vi "Simulation LV2G.vi"(6 "Operation (Get)":T1=enum."Get", 8 "error in (no error)":errorcluster, 11 "Simulation?":bool) -> (0 "error out":errorcluster, 3 "Simulation? out":bool)   [LabVIEW 2016]
uses:
  Typedefs/LV2G Operation.ctl
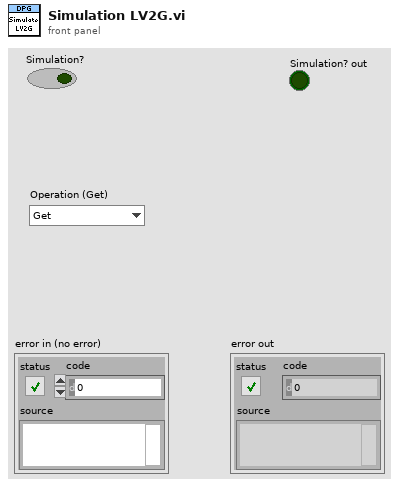
[diagram p1: front panel]
types:
  T1 = typedef "LV2G Operation.ctl" = enum16{"Initialize", "Set", "Get", "Close"}
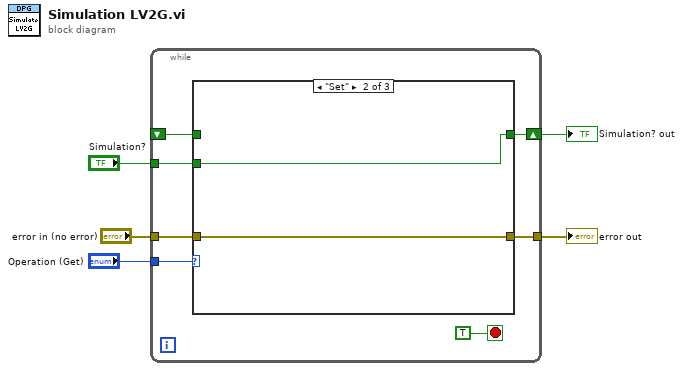
[diagram p0: block diagram]
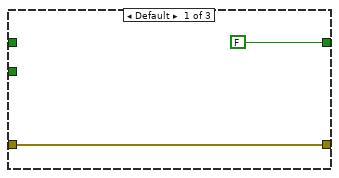
[diagram p2: hidden frame]
diagram:
  n1 = while {
    tunnel: "Operation (Get)" -> [w11]
    tunnel: "error in (no error)" -> [w10]
    tunnel: [w6] -> w4
    shift-right: [w9] -> w2
    shift-left: _ -> [w7]
    tunnel: "Simulation?" -> [w8]
    stop <- TRUE stop-if-true
    n2 = case shown="\"Set\"" w11 {
      tunnel: w10 -> [w13 w15 w17]
      tunnel: [FALSE ("Stop? out") w16 w18] -> w9
      tunnel: w8 -> [_ w16 _]
      tunnel: w7 -> [_ _ w18]
      tunnel: [w13 w15 w17] -> w6
      frame Default {
      }
      frame "Set" {
      }
      frame "Get" {
      }
    }
  }
  "error out" <- w4
  "Simulation? out" <- w2
